vi "Constructor.vi"(8 "error in (no error)":errorcluster, 10 "Table Name (Use Member Data)":string, 11 "Table Configuration in":refnum<class "Table Configuration.lvclass">) -> (0 "error out":errorcluster, 3 "Table Configuration out":refnum<class "Table Configuration.lvclass">)   [LabVIEW 2020, in "Table.lvlib" / "Table Configuration.lvclass"]
uses:
  Table Configuration.lvclass
  Table Configuration.lvclass/Table Configuration.ctl
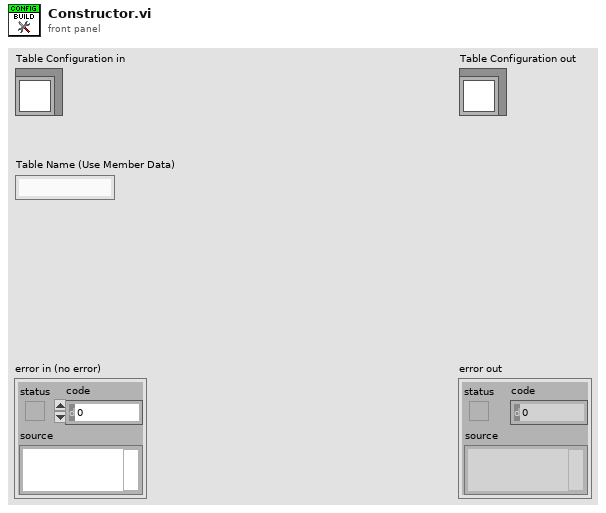
[diagram p1: front panel]
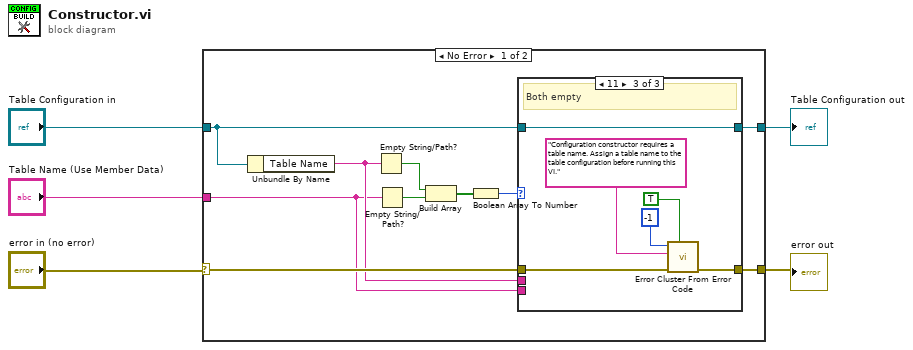
[diagram p0: block diagram]
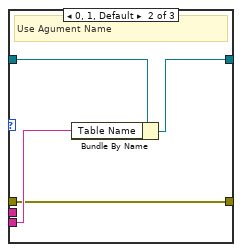
[diagram p3: hidden frame]
diagram:
  n1 = case shown="No Error" "error in (no error)" {
    selector: "error in (no error)" -> [w14 w29]
    tunnel: [w13 w29] -> w4
    tunnel: "Table Configuration in" -> [w12 w28]
    tunnel: [w15 w28] -> w2
    tunnel: "Table Name (Use Member Data)" -> [w7 _]
    frame No Error {
      n2 = Unbundle By Name(w12) -> ("Table Name"=w8:string)
      n3 = Empty String/Path?(string/path=w8) -> (empty?=w10:bool)
      n4 = Empty String/Path?(string/path=w7) -> (empty?=w9:bool)
      n5 = Build Array(w10, w9) -> (w11:bool[])
      n6 = Boolean Array To Number(Boolean array=w11) -> (number=w6:u32)
      n7 = case shown="11" w6 {
        tunnel: w12 -> [w16 w21 w27]
        tunnel: [w16 w20 w27] -> w15
        tunnel: w14 -> [w17 w18 w23]
        tunnel: [w17 w18 w22] -> w13
        tunnel: w8 -> [_ _ _]
        tunnel: w7 -> [_ w19 _]
        frame 2 {
          # "Member name OK"
        }
        frame 0, 1, Default {
          # "Use Agument Name"
          n8 = Bundle By Name(cluster=w21, "Table Name"=w19) -> (w20:refnum<class "Table Configuration.lvclass">)
        }
        frame 3 {
          # "Both empty"
          n9 = call <vilib>:"Error Cluster From Error Code.vi"("show call chain? (False)"=TRUE, "error in (no error)"=w23, "error message (\"\")"="Configuration constructor requires a table name. Assign a table name to the table configuration before running this VI.", "error code (0)"=-1) -> ("error out"=w22:errorcluster)  [unwired: 5 in]
        }
      }
    }
    frame Error {
    }
  }
  "error out" <- w4
  "Table Configuration out" <- w2
